vi "Step Counter.Start SubSection.vi"(1 "Step State":T1) -> (0 "Step State Out":T1)   [LabVIEW 2018]
uses:
  Step Counter.State Info.ctl
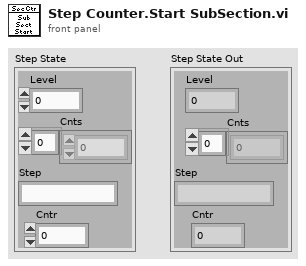
[diagram p1: front panel]
types:
  T1 = typedef "Step Counter.State Info.ctl" = cluster{"Level":i32, "Cnts":i32[], "Step":string, "Cntr":i32}
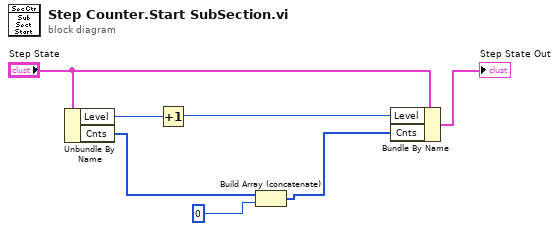
[diagram p0: block diagram]
diagram:
  n1 = Unbundle By Name("Step State") -> ("Level"=w7:i32, "Cnts"=w6:i32[])
  n2 = Increment(x=w7) -> (x+1=w3:i32)
  n3 = Build Array (concatenate)(w6, 0) -> (w4:i32[])
  n4 = Bundle By Name(cluster="Step State", "Level"=w3, "Cnts"=w4) -> (→"Step State Out":T1)
